vi "GFITS_PostProc.vi"(9 "logpath":path, 10 "log":bool, 11 "queue in":refnum<queue>) -> ()   [LabVIEW 2016]
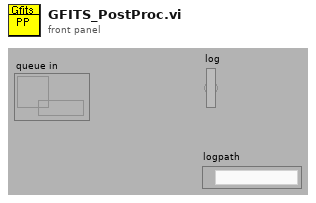
[diagram p1: front panel]
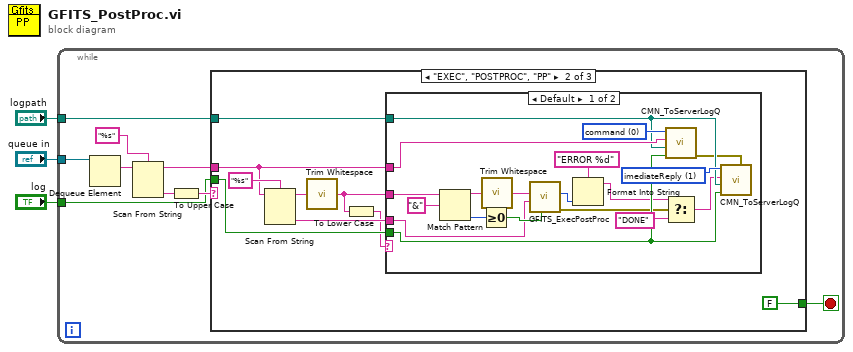
[diagram p0: block diagram]
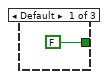
[diagram p2: hidden frame]
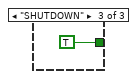
[diagram p4: hidden frame]
diagram:
  n1 = while {
    tunnel: "queue in" -> [w12]
    tunnel: "logpath" -> [w5]
    tunnel: "log" -> [w4]
    stop <- w7 stop-if-true
    n2 = Dequeue Element(queue=w12) -> (element=w11:string)  [unwired: 1 in, 4 out]
    n3 = Scan From String(format string="%s", input string=w11) -> (remaining string=w8:string, output 1=w9:string)  [unwired: 2 in, 3 out]
    n4 = To Upper Case(1:w9) -> (0:w6:string)
    n5 = case shown="\"EXEC\", \"POSTPROC\", \"PP\"" w6 {
      tunnel: w8 -> [_ w16 _]
      tunnel: [FALSE FALSE TRUE] -> w7
      tunnel: w5 -> [_ w18 _]
      tunnel: w4 -> [_ w17 _]
      frame Default {
      }
      frame "EXEC", "POSTPROC", "PP" {
        n6 = Scan From String(format string="%s", input string=w16) -> (remaining string=w20:string, output 1=w19:string)  [unwired: 2 in, 3 out]
        n7 = call <vilib>:"Trim Whitespace.vi"("string"=w20) -> ("trimmed string"=w15:string)  [unwired: 1 in]
        n8 = To Lower Case(string=w15) -> (all lower case string=w14:string)
        n9 = case shown="Default" w14 {
          tunnel: w19 -> [w36 _]
          tunnel: w15 -> [w41 _]
          tunnel: w18 -> [w30 _]
          tunnel: w17 -> [w31 _]
          tunnel: w16 -> [w35 _]
          frame Default {
            w32 = u16 1 items=["command", "imediateReply", "Callback Reply", "Information", "none"] ("type")
            w34 = u16 0 items=["command", "imediateReply", "Callback Reply", "Information", "none"] ("type")
            n10 = Match Pattern(string=w41, regular expression="&") -> (before substring=w37:string, offset past match=w39:i32)  [unwired: 3 out]
            n11 = Greater Or Equal To 0?(x=w39) -> (x >= 0?=w38:bool)
            n12 = call <vilib>:"Trim Whitespace.vi"("string"=w37) -> ("trimmed string"=w33:string)  [unwired: 1 in]
            n13 = call "GFITS_ExecPostProc.vi"("background"=w38, "impath"=w36, "postproc"=w33) -> ("error out"=w29:errorcluster, "return type"=w25:i32)  [unwired: 2 in, 5 out]
            n14 = Format Into String(format string="ERROR %d", w25) -> (resulting string=w24:string)  [unwired: 2 in, 1 out]
            n15 = call "CMN_ToServerLogQ.vi"("Log"=w31, "file"=w30, "string"=w35, "type"=w34) -> ("error out"=w23:errorcluster)  [unwired: 2 in, 4 out]
            n16 = Select(t=w24, s=w29, f="DONE") -> (s? t:f=w27:string)
            n17 = call "CMN_ToServerLogQ.vi"("error in (no error)"=w23, "Log"=w31, "file"=w30, "string"=w27, "type"=w32) -> ()  [unwired: 1 in, 5 out]
          }
          frame "", "none" {
          }
        }
      }
      frame "SHUTDOWN" {
      }
    }
  }
